vi "Get System Stats.vi"(8 "Error In":errorcluster) -> (0 "error out":errorcluster, 3 "System Info":T1 {"Calendar"."AlgorithmType" items=["Unknown", "SolarCalendar", "LunarCalendar", "LunisolarCalendar"]})   [LabVIEW 2017]
uses:
  controls/System_Info.ctl
  controls/System_Spec.ctl
  controls/System_Calendar.ctl
  controls/System_NumberFormats.ctl
  Microsoft.VisualBasic
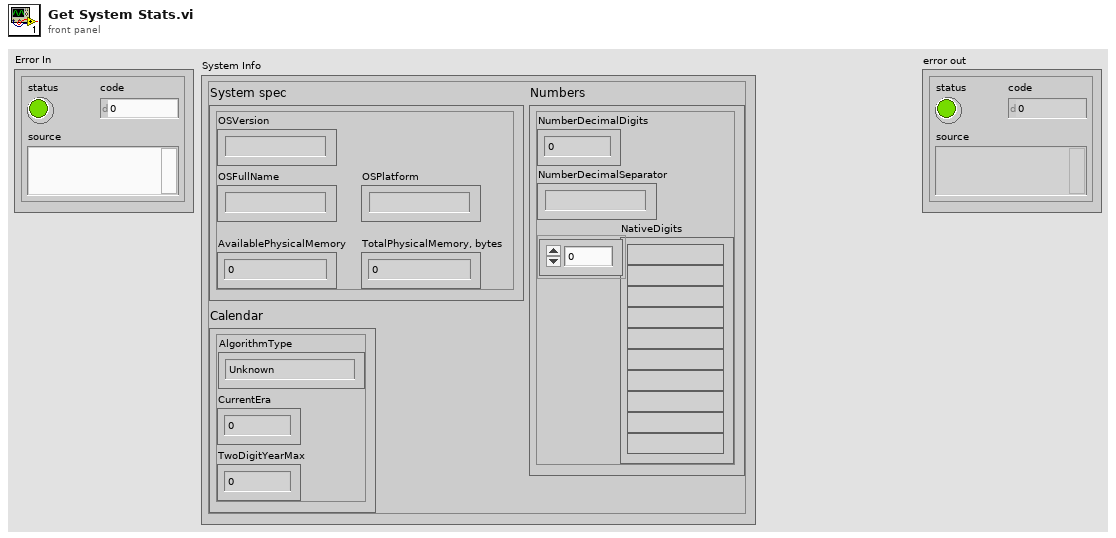
[diagram p1: front panel]
types:
  T1 = typedef "System_Info.ctl" = cluster{"System spec":T2, "Calendar":T3, "Numbers":T4}
  T2 = typedef "System_Spec.ctl" = cluster{"OSVersion":string, "OSFullName":string, "OSPlatform":string, "AvailablePhysicalMemory":u64, "TotalPhysicalMemory, bytes":u64}
  T3 = typedef "System_Calendar.ctl" = cluster{"AlgorithmType":i32, "CurrentEra":i32, "TwoDigitYearMax":i32}
  T4 = typedef "System_NumberFormats.ctl" = cluster{"NumberDecimalDigits":i32, "NumberDecimalSeparator":string, "NativeDigits":string[]}
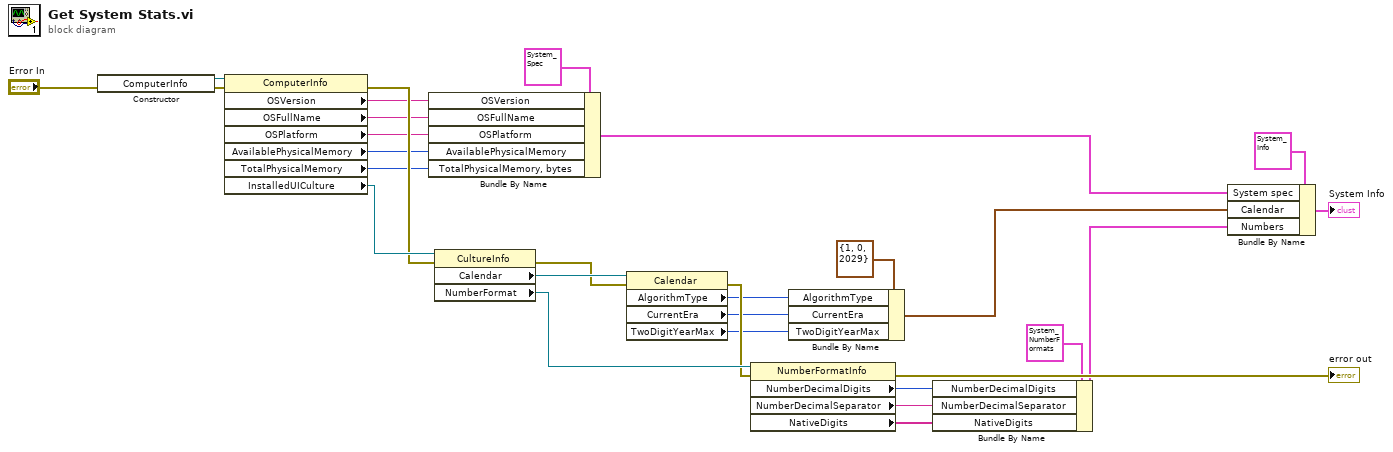
[diagram p0: block diagram]
diagram:
  n1 = constructor class="ComputerInfo"(error in="Error In") -> (reference out=w29:refnum<k24>, error out=w28:errorcluster)  [unwired: 2 in, 1 out]
  n2 = property class="ComputerInfo"(reference=w29, error in=w28) -> (error out=w24:errorcluster, "OSVersion"=w11:string, "OSFullName"=w10:string, "OSPlatform"=w9:string, "AvailablePhysicalMemory"=w8:u64, "TotalPhysicalMemory"=w7:u64, "InstalledUICulture"=w27:refnum<k24>)  [unwired: 1 out]
  n3 = Bundle By Name(cluster=T2 {"OSVersion"="6.1.7601.65536", "OSFullName"="Microsoft Windows 7 Ultimate ", "OSPlatform"="Win32NT", "AvailablePhysicalMemory"=8140726272, "TotalPhysicalMemory, bytes"=16868524032} ("System spec"), "OSVersion"=w11, "OSFullName"=w10, "OSPlatform"=w9, "AvailablePhysicalMemory"=w8, "TotalPhysicalMemory, bytes"=w7) -> (w14:T2)
  n4 = property class="CultureInfo"(reference=w27, error in=w24) -> (error out=w25:errorcluster, "Calendar"=w26:refnum<k24>, "NumberFormat"=w23:refnum<k24>)  [unwired: 1 out]
  n5 = property class="Calendar"(reference=w26, error in=w25) -> (error out=w20:errorcluster, "AlgorithmType"=w1:i32, "CurrentEra"=w2:i32, "TwoDigitYearMax"=w3:i32)  [unwired: 1 out]
  n6 = property class="NumberFormatInfo"(reference=w23, error in=w20) -> (error out=→"error out":errorcluster, "NumberDecimalDigits"=w4:i32, "NumberDecimalSeparator"=w5:string, "NativeDigits"=w6:string[])  [unwired: 1 out]
  n7 = Bundle By Name(cluster=T3 {"AlgorithmType"=1, "CurrentEra"=0, "TwoDigitYearMax"=2029} ("Calendar"), "AlgorithmType"=w1, "CurrentEra"=w2, "TwoDigitYearMax"=w3) -> (w13:T3)
  n8 = Bundle By Name(cluster=T4 {"NumberDecimalDigits"=2, "NumberDecimalSeparator"=",", "NativeDigits"=["0", "1", "2", "3", "4", "5", "6", "7", "8", "9"]} ("Numbers"), "NumberDecimalDigits"=w4, "NumberDecimalSeparator"=w5, "NativeDigits"=w6) -> (w12:T4)
  n9 = Bundle By Name(cluster=T1 {"System spec"={"OSVersion"="", "OSFullName"="", "OSPlatform"="", "AvailablePhysicalMemory"=0, "TotalPhysicalMemory, bytes"=0}, "Calendar"={"AlgorithmType"=0, "CurrentEra"=0, "TwoDigitYearMax"=0}, "Numbers"={"NumberDecimalDigits"=0, "NumberDecimalSeparator"="", "NativeDigits"=[]}} ("System Info 2"), "System spec"=w14, "Calendar"=w13, "Numbers"=w12) -> (→"System Info":T1)
